vi "test_Bitfile Reload_Group Scalars Data Type Change.vi"(8 "error in (no error)":errorcluster, 11 "TestCase in":refnum<class "FPGA Addon Bitfile Reload Unit Tests.lvclass">=refnum) -> (0 "error out":errorcluster, 3 "TestCase out":refnum<class "FPGA Addon Bitfile Reload Unit Tests.lvclass">)   [LabVIEW 2026, in "FPGA Addon Bitfile Reload Unit Tests.lvclass"]
uses:
  FPGA Addon Bitfile Reload Unit Tests.lvclass
  APIs/Scripting API/TypeDefs/Output Scalar Data.ctl
  APIs/Scripting API/Scripting API.lvlib
  FPGA Addon Test Class/FPGA Addon Test Class.lvclass
  Addon/Addon System Explorer/FPGA Addon System Explorer.lvlib
  APIs/Scripting API/Public/Bitfile Resources/Import Bitfile Scalars (Instances)/Import Scalars - all.vi
  Addon/Addon Shared/Types/FPGA Addon Data Type.ctl
  Addon/Addon Shared/FPGA Addon Shared.lvlib
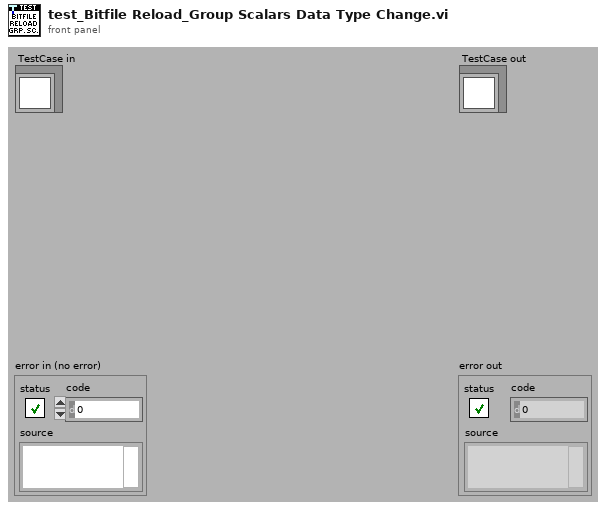
[diagram p1: front panel]
types:
  T1 = typedef "Scripting API.lvlib/Output Scalar Data.ctl" = cluster{"Bitfile Name":string, "SysDef Channel Name":string, "Imported":bool, "Data Type":T2}
  T2 = typedef "FPGA Addon Shared.lvlib/FPGA Addon Data Type.ctl" = enum8{"<Null>", "I8", "I16", "I32", "I64", "U8", "U16", "U32", "U64", "SGL", "Boolean", "Analog PWM In Settings", "Analog PWM In", "Digital PWM In Settings", "Digital PWM In", "Digital PWM Out", "Sine Out", "FXP", "FXP+/-24.5", "FXP+/-16.5", "FXP+/-32.8", "FXP+/-64.32", "FXP+/-16.7", "FXP+/-20.5", "FXP+/-27.5", "FXP+/-32.16", "FXP+16.3", "FXP+18.3", "Digital Static In", "Digital Static Out", "Digital Static In Settings", "Digital WSS Out", "Quad Encoder Settings", "Quad Encoder In", "Group"}
  T3 = typedef "Custom Device API.lvlib/Custom Device Item Ref.ctl" = u64
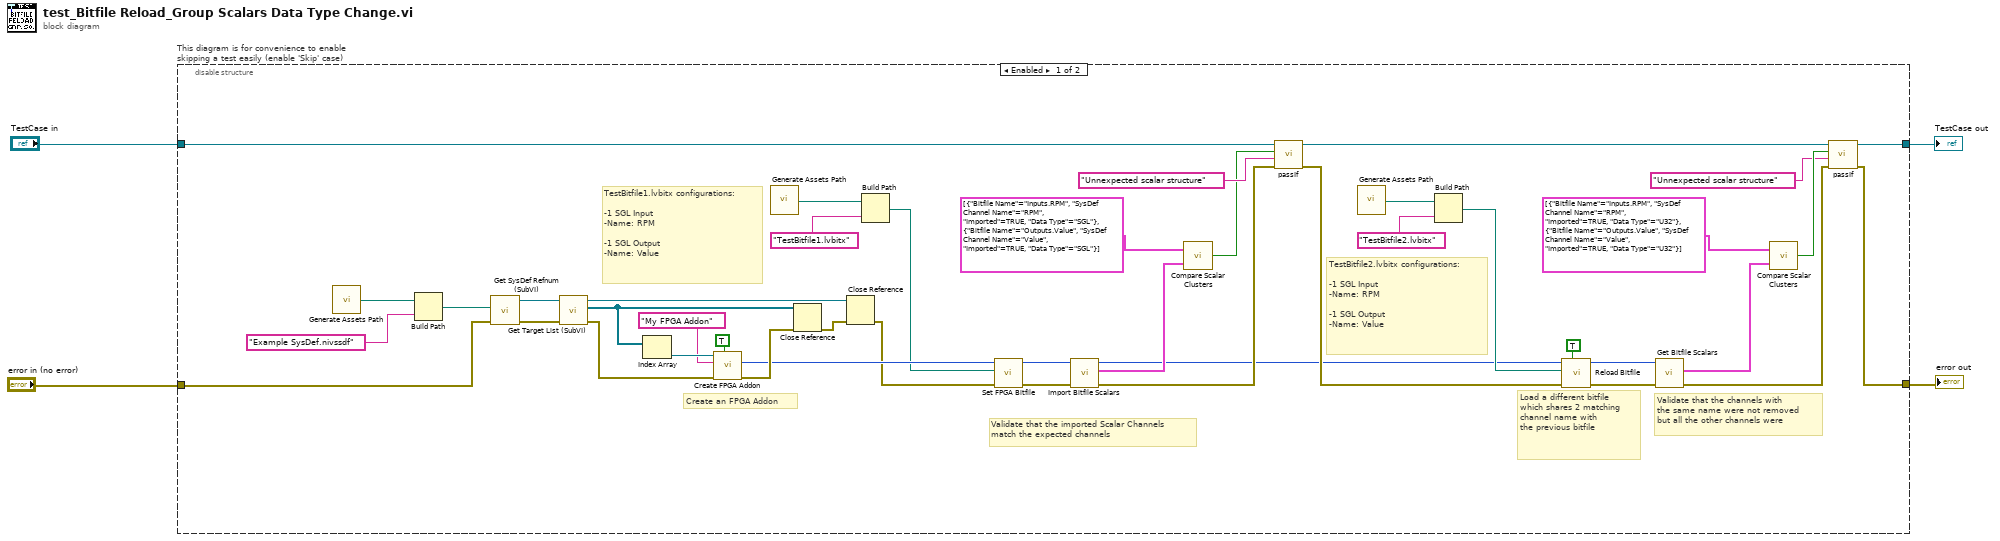
[diagram p0: block diagram]
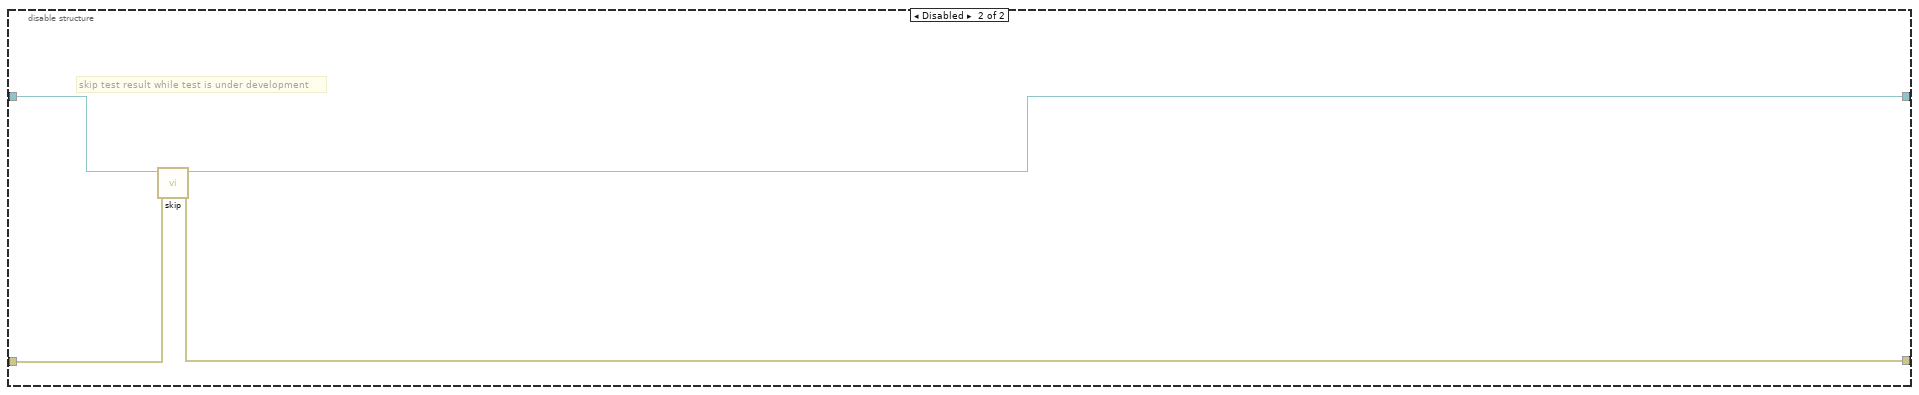
[diagram p2: hidden frame]
diagram:
  n1 = disable-structure "This diagram is for convenience to enable skipping a test easily (enable 'Skip' case)" shown="Enabled" {
    disable-tunnel: "TestCase in" -> [w11 w51]
    disable-tunnel: [w9 w49] -> w1
    disable-tunnel: [w8 w50] -> w3
    disable-tunnel: "error in (no error)" -> [w10 w48]
    frame Enabled {
      # "TestBitfile2.lvbitx configurations:\n\n-1 SGL Input\n-Name: RPM\n\n-1 SGL Output\n-Name: Value"
      # "TestBitfile1.lvbitx configurations:\n\n-1 SGL Input\n-Name: RPM\n\n-1 SGL Output\n-Name: Value"
      # "Validate that the channels with \nthe same name were not removed\nbut all the other channels were"
      # "Load a different bitfile\nwhich shares 2 matching\nchannel name with \nthe previous bitfile"
      # "Validate that the imported Scalar Channels\nmatch the expected channels"
      # "Create an FPGA Addon"
      n2 = call "Generate Assets Path.vi"() -> ("Assets path"=w27:path)
      n3 = Build Path(base path=w27, name or relative path="Example SysDef.nivssdf") -> (appended path=w46:path)
      n4 = call "Get SysDef Refnum (SubVI).vi"("error in (no error)"=w10, "System Definition path"=w46) -> ("error out"=w42:errorcluster, "NationalInstruments.VeriStand.SystemDefinitionAPI.SystemDefinition"=w45:refnum<k39>)  [unwired: 8 in]
      n5 = call "Get Target List (SubVI).vi"("error in (no error)"=w42, "NationalInstruments.VeriStand.SystemDefinitionAPI.SystemDefinition"=w45) -> ("error out"=w41:errorcluster, "Target List Refnums"=w40:refnum<k39>[], "NationalInstruments.VeriStand.SystemDefinitionAPI.SystemDefinition"=w39:refnum<k39>)  [unwired: 7 in]
      n6 = Index Array(array=w40) -> (element=w44:refnum<k39>)  [unwired: 1 in]
      n7 = call "Create FPGA Addon.vi"("group scalars"=TRUE, "error in"=w41, "FPGA addon name"="My FPGA Addon", "NationalInstruments.VeriStand.SystemDefinitionAPI.Target"=w44) -> ("error out"=w37:errorcluster, "FPGA addon refnum"=w35:T3)  [unwired: 5 in, 1 out]
      n8 = call "Generate Assets Path.vi"() -> ("Assets path"=w26:path)
      n9 = Close Reference(reference=w40, error in (no error)=w37) -> (error out=w38:errorcluster)
      n10 = Close Reference(reference=w39, error in (no error)=w38) -> (error out=w34:errorcluster)
      n11 = Build Path(base path=w26, name or relative path="TestBitfile1.lvbitx") -> (appended path=w32:path)
      n12 = call "Set FPGA Bitfile.vi"("error in"=w34, "FPGA bitfile path"=w32, "FPGA addon refnum in"=w35) -> ("error out"=w31:errorcluster, "FPGA addon refnum out"=w30:T3)  [unwired: 7 in]
      n13 = call-poly "Import Bitfile Scalars.vi"("error in"=w31, "FPGA addon refnum in"=w30) -> ("error out"=w29:errorcluster, "imported bitfile scalars out"=w24:T1[], "FPGA addon refnum out"=w19:T3)  [unwired: 7 in]
      n14 = call "Compare Scalar Clusters.vi"("Target bitfile scalars in"=w24, "Reference bitfile scalars in"=T1[] [{"Bitfile Name"="Inputs.RPM", "SysDef Channel Name"="RPM", "Imported"=TRUE, "Data Type"=enum."SGL"}, {"Bitfile Name"="Outputs.Value", "SysDef Channel Name"="Value", "Imported"=TRUE, "Data Type"=enum."SGL"}] ("imported bitfile scalars out")) -> ("Equal ?"=w25:bool)
      n15 = call-dynamic "passIf.vi"("error in (no error)"=w29, "message (\"\")"="Unnexpected scalar structure" ("message (\"\")"), "pass"=w25, "TestCase in"=w11) -> ("error out"=w21:errorcluster, "TestCase out"=w16:refnum<class "FPGA Addon Bitfile Reload Unit Tests.lvclass">)  [unwired: 6 in]
      n16 = call "Generate Assets Path.vi"() -> ("Assets path"=w22:path)
      n17 = Build Path(base path=w22, name or relative path="TestBitfile2.lvbitx") -> (appended path=w20:path)
      n18 = call "Reload Bitfile.vi"("Group"=TRUE, "error in (no error)"=w21, "NewVal"=w20, "Item Ref in"=w19) -> ("error out"=w18:errorcluster, "Section Ref out"=w17:T3)  [unwired: 6 in]
      n19 = call "Get Bitfile Scalars.vi"("error in"=w18, "FPGA addon refnum in"=w17) -> ("error out"=w14:errorcluster, "bitfile scalars out"=w15:T1[])  [unwired: 7 in, 1 out]
      n20 = call "Compare Scalar Clusters.vi"("Target bitfile scalars in"=w15, "Reference bitfile scalars in"=T1[] [{"Bitfile Name"="Inputs.RPM", "SysDef Channel Name"="RPM", "Imported"=TRUE, "Data Type"=enum."U32"}, {"Bitfile Name"="Outputs.Value", "SysDef Channel Name"="Value", "Imported"=TRUE, "Data Type"=enum."U32"}] ("imported bitfile scalars out")) -> ("Equal ?"=w13:bool)
      n21 = call-dynamic "passIf.vi"("error in (no error)"=w14, "message (\"\")"="Unnexpected scalar structure" ("message (\"\")"), "pass"=w13, "TestCase in"=w16) -> ("error out"=w8:errorcluster, "TestCase out"=w9:refnum<class "FPGA Addon Bitfile Reload Unit Tests.lvclass">)  [unwired: 6 in]
    }
    frame Disabled {
      # "skip test result while test is under development"
      n22 = call <vilib>:"skip.vi"("error in (no error)"=w48, "TestCase in"=w51) -> ("error out"=w50:errorcluster, "TestCase out"=w49:refnum<class "FPGA Addon Bitfile Reload Unit Tests.lvclass">)  [unwired: 8 in]
    }
  }
  "error out" <- w3
  "TestCase out" <- w1
